vi "search_comm_map_for_Var.vi"(10 "Parameter":string, 11 "Comm variable definitions":T1[](array[typedef]) {"Cluster"."Mode" items=["None", "MODBUS", "HART", "Profibus DP", "Profibus PA", "Fieldbus", "DeviceNET"]}) -> (2 "found?":bool, 3 "index":i32)   [LabVIEW 2016]
uses:
  Typedef/comm_variable_definition.ctl
  Typedef/Comm_mode_and_address_type.ctl
  Typedef/Comm_mode_type_combo.ctl
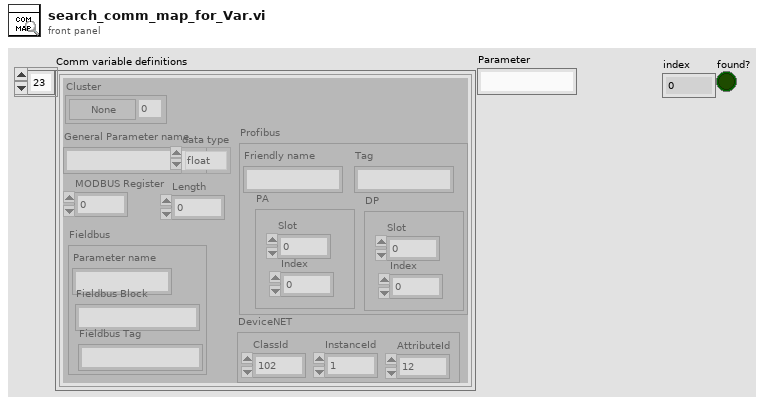
[diagram p1: front panel]
types:
  T1 = typedef "comm_variable_definition.ctl" = cluster{"General Parameter name":string, "MODBUS Register":i32, "Profibus":cluster{"Friendly name":string, "PA":cluster{"Slot":i32, "Index":i32}, "DP":cluster{"Slot":i32, "Index":i32}, "Tag":string}, "Fieldbus":cluster{"Parameter name":string, "Fieldbus Block":string, "Fieldbus Tag":string}, "data type":enum16{"float", "UINT", "UINT32", "STRING"}, "DeviceNET":cluster{"ClassId":u16, "InstanceId":u16, "AttributeId":u8}, "Cluster":T2, "Length":i32}
  T2 = typedef "Comm_mode_and_address_type.ctl" = cluster{"address":i32, "Mode":T3}
  T3 = typedef "Comm_mode_type_combo.ctl" = u16
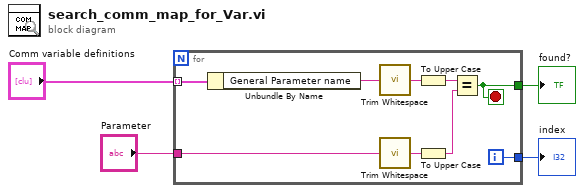
[diagram p0: block diagram]
diagram:
  n1 = for {
    tunnel: "Comm variable definitions" -> [w13] mode=indexing
    tunnel: "Parameter" -> [w11]
    tunnel: [w8] -> w2
    tunnel: [w7] -> w1
    i -> [w8]
    stop <- w7 stop-if-true
    n2 = Unbundle By Name(w13) -> ("General Parameter name"=w12:string)
    n3 = call <vilib>:"Trim Whitespace.vi"("string"=w12) -> ("trimmed string"=w5:string)  [unwired: 1 in]
    n4 = call <vilib>:"Trim Whitespace.vi"("string"=w11) -> ("trimmed string"=w6:string)  [unwired: 1 in]
    n5 = To Upper Case(1:w5) -> (0:w10:string)
    n6 = To Upper Case(1:w6) -> (0:w9:string)
    n7 = Equal?(x=w10, y=w9) -> (x = y?=w7:bool)
  }
  "index" <- w2
  "found?" <- w1
